vi "queue driver.vi"(0 "Enqueue":string[](array[string]), 2 "Name":string, 11 "Error in":errorcluster, 13 "Queue operations":T1) -> (4 "Dequeued element":string, 15 "Error out":errorcluster)   [LabVIEW 2020, in "coffee machine.lvlib"]
uses:
  coffee machine.lvlib
  Typedefs/Queue operations.ctl
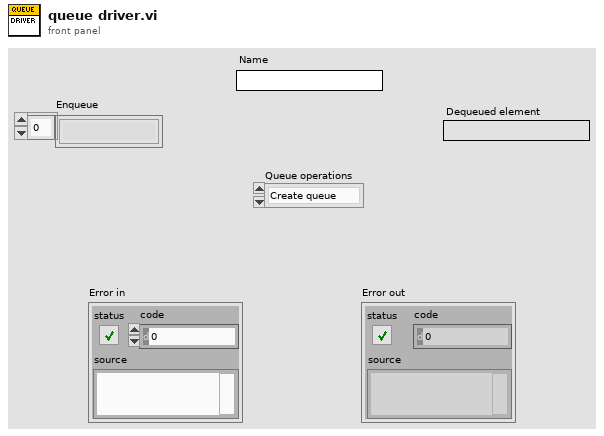
[diagram p1: front panel]
types:
  T1 = typedef "coffee machine.lvlib/Queue operations.ctl" = enum16{"Create queue", " Enqueue N", "Enstack N", "Dequeue", "Flush", "Release", ""}
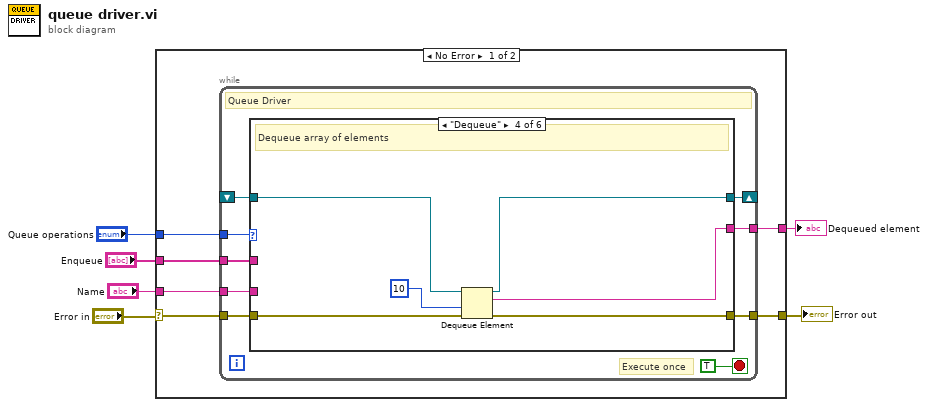
[diagram p0: block diagram]
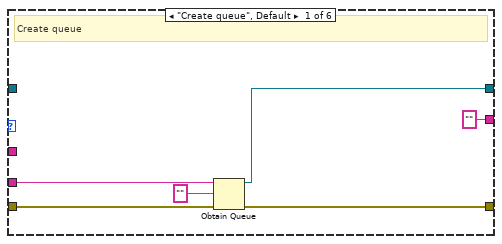
[diagram p2: hidden frame]
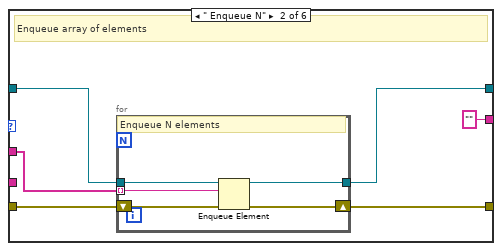
[diagram p3: hidden frame]
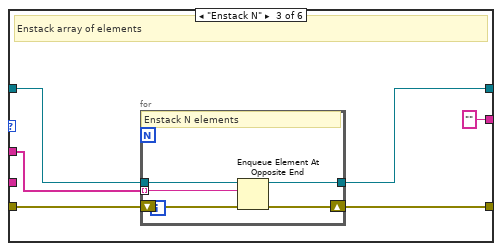
[diagram p4: hidden frame]
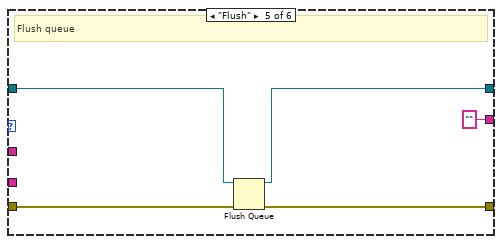
[diagram p5: hidden frame]
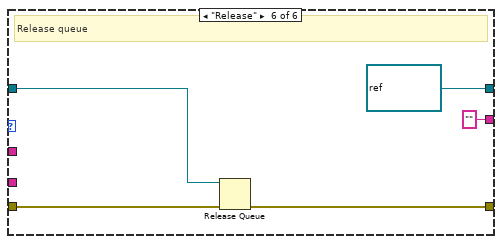
[diagram p6: hidden frame]
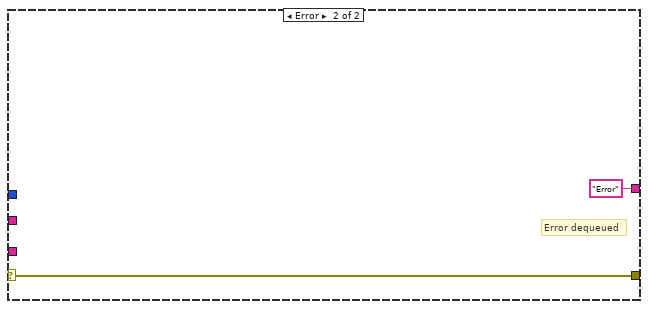
[diagram p7: hidden frame]
diagram:
  n1 = case shown="No Error" "Error in" {
    selector: "Error in" -> [w11 w67]
    tunnel: "Queue operations" -> [w12 _]
    tunnel: [w10 w67] -> w4
    tunnel: "Name" -> [w9 _]
    tunnel: "Enqueue" -> [w8 _]
    tunnel: [w7 "Error"] -> w1
    frame No Error {
      n2 = while {
        tunnel: w12 -> [w20]
        tunnel: w11 -> [w19]
        tunnel: [w18] -> w10
        tunnel: w9 -> [w17]
        shift-right: [w16] -> _
        shift-left: _ -> [w15]
        tunnel: w8 -> [w14]
        tunnel: [w13] -> w7
        stop <- TRUE stop-if-true
        # "Execute once"
        # "Queue Driver"
        n3 = case shown="\"Dequeue\"" w20 {
          tunnel: w19 -> [w27 w33 w44 w55 w60 w65]
          tunnel: [w26 w32 w43 w54 w59 w64] -> w18
          tunnel: w17 -> [w25 _ _ _ _ _]
          tunnel: [w24 w30 w41 w52 w57 refnum<queue> refnum ("queue out")] -> w16
          tunnel: w15 -> [_ w31 w42 w53 w58 w63]
          tunnel: w14 -> [_ w29 w40 _ _ _]
          tunnel: ["" "" "" w50 "" ""] -> w13
          frame "Create queue", Default {
            # "Create queue"
            n4 = Obtain Queue(name (unnamed)=w25, element data type="", error in (no error)=w27) -> (queue out=w24:refnum<queue>, error out=w26:errorcluster)  [unwired: 2 in, 1 out]
          }
          frame " Enqueue N" {
            # "Enqueue array of elements"
            n5 = for {
              tunnel: w31 -> [w36]
              tunnel: [w35] -> w30
              shift-right: [w37] -> w32
              shift-left: w33 -> [w38]
              tunnel: w29 -> [w34] mode=indexing
              # "Enqueue N elements"
              n6 = Enqueue Element(queue=w36, element=w34, error in (no error)=w38) -> (queue out=w35:refnum<queue>, error out=w37:errorcluster)  [unwired: 1 in, 1 out]
            }
          }
          frame "Enstack N" {
            # "Enstack array of elements"
            n7 = for {
              tunnel: w42 -> [w47]
              tunnel: [w46] -> w41
              shift-right: [w48] -> w43
              shift-left: w44 -> [w49]
              tunnel: w40 -> [w45] mode=indexing
              # "Enstack N elements"
              n8 = Enqueue Element At Opposite End(queue=w47, element=w45, error in (no error)=w49) -> (queue out=w46:refnum<queue>, error out=w48:errorcluster)  [unwired: 1 in, 1 out]
            }
          }
          frame "Dequeue" {
            # "Dequeue array of elements"
            n9 = Dequeue Element(queue=w53, timeout in ms (-1)=10, error in (no error)=w55) -> (queue out=w52:refnum<queue>, element=w50:string, error out=w54:errorcluster)  [unwired: 1 out]
          }
          frame "Flush" {
            # "Flush queue"
            n10 = Flush Queue(queue=w58, error in (no error)=w60) -> (queue out=w57:refnum<queue>, error out=w59:errorcluster)  [unwired: 1 out]
          }
          frame "Release" {
            # "Release queue"
            n11 = Release Queue(queue=w63, error in (no error)=w65) -> (error out=w64:errorcluster)  [unwired: 1 in, 2 out]
          }
        }
      }
    }
    frame Error {
      # "Error dequeued"
    }
  }
  "Error out" <- w4
  "Dequeued element" <- w1
